vi "lvssh2_session_callback_send_handler_64.vi"(4 "lvssh2_session_callback_send":refnum<vi>, 5 "Event Data":T1, 6 "User Event Ref":refnum<user-event>, 7 "Event Common Data":T3 {"Event Source" items=["LabVIEW UI"=0, "ActiveX"=1, "User Event"=25]}) -> ()   [LabVIEW 2017, in "libssh2.lvlib"]
uses:
  libssh2.lvlib
  <vilib>/event_ctls.llb/eventsource.ctl
  lvssh2_session_callback_send_function_input_args_64.ctl
  lvssh2_extensions_64.dll
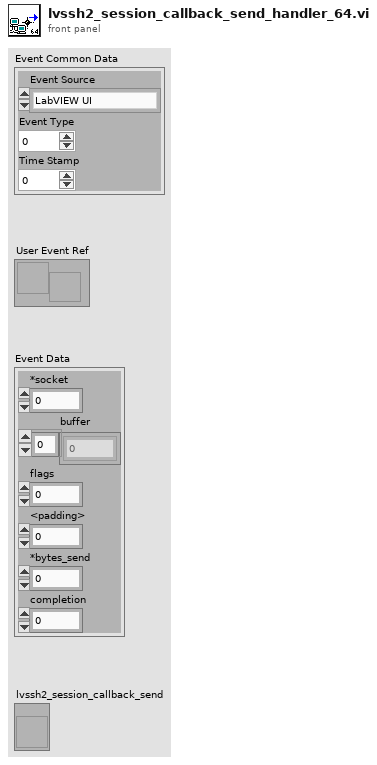
[diagram p1: front panel]
types:
  T1 = typedef "libssh2.lvlib/lvssh2_session_callback_send_function_input_args_64.ctl" = cluster{"*socket":u64, "buffer":u8[], "flags":i32, "<padding>":i32, "*bytes_send":u64, "completion":u64}
  T2 = typedef "eventsource.ctl" = u32
  T3 = cluster{"Event Source":T2, "Event Type":u32, "Time Stamp":u32}
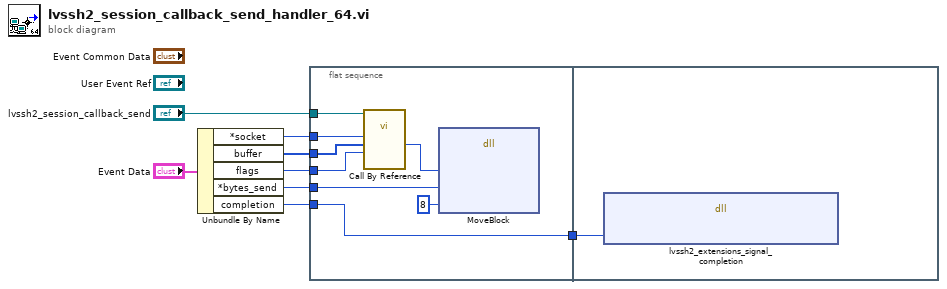
[diagram p0: block diagram]
diagram:
  n1 = Unbundle By Name("Event Data") -> ("*socket"=w6:u64, "buffer"=w4:u8[], "flags"=w5:i32, "*bytes_send"=w3:u64, "completion"=w2:u64)
  n2 = flat-sequence {
    tunnel: "lvssh2_session_callback_send" -> [w16]
    tunnel: w6 -> [w15]
    tunnel: w5 -> [w14]
    tunnel: w4 -> [w13]
    tunnel: w3 -> [w11]
    tunnel: w2 -> [w9]
    tunnel: [w9] -> w1
    tunnel: w1 -> [w17]
    frame #0 {
      n3 = call-by-ref "?"(reference=w16, "flags"=w14, "buffer"=w13, "socket"=w15) -> ("bytes send"=w12:i64)  [unwired: 8 in, 3 out]
      n4 = dll-call lib="LabVIEW" fn="MoveBlock"("ps"=w12, "pd"=w11, "size"=u64 8) -> ()  [unwired: 7 in, 2 out]
    }
    frame #1 {
      n5 = dll-call lib="C:/Users/pasca/Projects/Home/lvssh2/libssh2/lvssh2_extensions**.*" fn="lvssh2_extensions_signal_completion"("completion"=w17) -> ()  [unwired: 5 in, 2 out]
    }
  }
